vi "New.vi"(8 "error in (no error)":errorcluster, 11 "BCAdmin":refnum<class "BCAdmin.lvclass">) -> (0 "error out":errorcluster, 1 "BC ID":i32, 2 "First?":bool, 3 "BCAdmin":refnum<class "BCAdmin.lvclass">)   [LabVIEW 2014, in "BusController.lvlib" / "BCAdmin.lvclass"]
uses:
  BCAdmin.lvclass
  BCAdmin.lvclass/BCAdmin.ctl
  Accessors/Read BCRegRef.vi
  Accessors/Read BC ID.vi
  Accessors/Write BCRegRef.vi
  Accessors/Write First_.vi
  Registry/BCReg.lvclass
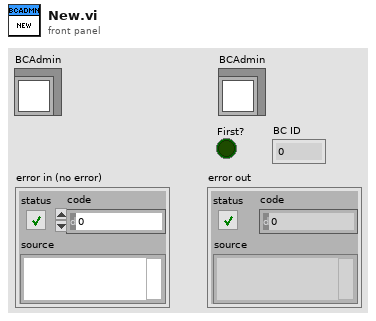
[diagram p1: front panel]
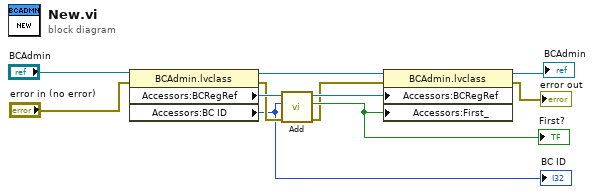
[diagram p0: block diagram]
diagram:
  n1 = property class="BCAdmin.lvclass"(reference="BCAdmin", error in="error in (no error)") -> (reference out=w9:refnum<class "BCAdmin.lvclass">, error out=w7:errorcluster, "Accessors:BCRegRef"=w10:refnum<data-value>, "Accessors:BC ID"=w6:i32)
  "BC ID" <- w6
  n2 = call "Add.vi"("error in (no error)"=w7, "BC ID"=w6, "BCReg"=w10) -> ("error out"=w3:errorcluster, "First?"=w4:bool, "BCReg"=w5:refnum<data-value>)  [unwired: 6 in]
  "First?" <- w4
  n3 = property class="BCAdmin.lvclass"(reference=w9, error in=w3, "Accessors:BCRegRef"=w5, "Accessors:First_"=w4) -> (reference out=→"BCAdmin":refnum<class "BCAdmin.lvclass">, error out=→"error out":errorcluster)
